vi "Set Debug.vi"(10 "Debug":bool, 11 "Module in":refnum<class "Module.lvclass">) -> (3 "Module out":refnum<class "Module.lvclass">)   [LabVIEW 2020, in "Volatus.lvlib" / "Module.lvclass"]
uses:
  Module.lvclass
  Module.lvclass/Module.ctl
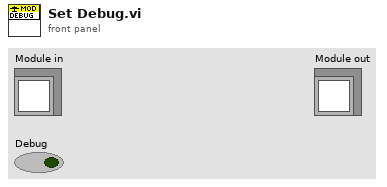
[diagram p1: front panel]
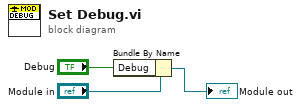
[diagram p0: block diagram]
diagram:
  n1 = Bundle By Name(cluster="Module in", "Debug"="Debug") -> (→"Module out":refnum<class "Module.lvclass">)
